vi "FTW-Endpoint-Multipart-Reply.vi"(0 "FTW Endpoint":refnum<class "FTW-Endpoint-TCP.lvclass">, 5 "Multipart Message":string[](array[string]), 7 "Timeout":i32 format="%dmsec", 11 "error in":errorcluster) -> (4 "FTW Endpoint out":refnum<class "FTW-Endpoint-TCP.lvclass">, 6 "Timed out?":bool, 15 "error out":errorcluster)   [LabVIEW 2013, in "FTW-Endpoint-TCP.lvclass"]
uses:
  FTW-Endpoint-TCP.lvclass
  FTW-Endpoint-TCP.lvclass/FTW-Endpoint-TCP.ctl
  Core/src/Error/FTW-ERR-Clear.vi
panel:
  # "Inputs"
  # "Outputs"
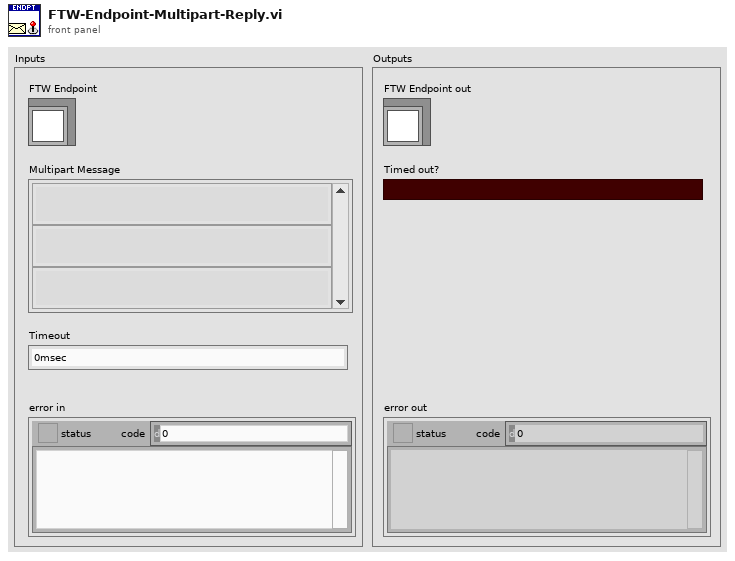
[diagram p1: front panel]
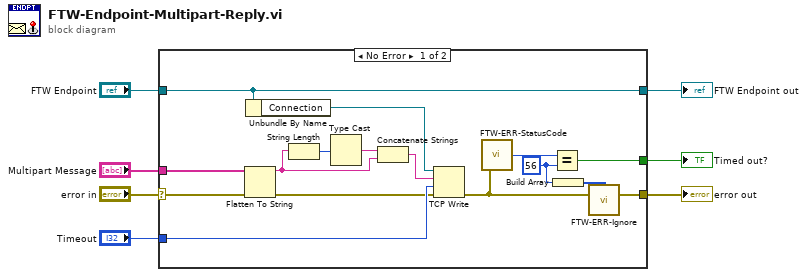
[diagram p0: block diagram]
diagram:
  n1 = case shown="No Error" "error in" {
    selector: "error in" -> [w21 w25]
    tunnel: [w10 w25] -> w6
    tunnel: [w22 w24] -> w4
    tunnel: "FTW Endpoint" -> [w22 w24]
    tunnel: "Multipart Message" -> [w12 _]
    tunnel: [w11 _] -> w5
    tunnel: "Timeout" -> [w23 _]
    frame No Error {
      w9 = 56 ("x")
      n2 = Flatten To String(anything=w12, error in (no error)=w21) -> (data string=w13:string, error out=w20:errorcluster)  [unwired: 2 in, 1 out]
      n3 = Unbundle By Name(w22) -> ("Connection"=w19:refnum<k5>)
      n4 = String Length(string=w13) -> (length=w16:i32)
      n5 = Type Cast(x=w16) -> (*(type *) &x=w15:string)  [unwired: 1 in]
      n6 = Concatenate Strings(w15, w13) -> (w14:string)
      n7 = TCP Write(connection ID=w19, data in=w14, error in (no error)=w20, 9:w23) -> (error out=w18:errorcluster)  [unwired: 2 out]
      n8 = call "FTW-ERR-StatusCode.vi"("error to check"=w18) -> ("Code"=w17:i32)
      n9 = Equal?(x=w17, y=w9) -> (x = y?=w11:bool)
      n10 = Build Array(w9) -> (w8:i32[])
      n11 = call "FTW-ERR-Ignore.vi"("Codes to filter"=w8, "error to filter"=w18) -> ("filtered error"=w10:errorcluster)  [unwired: 13 in]
    }
    frame Error {
    }
  }
  "error out" <- w6
  "FTW Endpoint out" <- w4
  "Timed out?" <- w5
